vi "show_message.vi"(6 "display time (ms)":i32=5000, 7 "Icon (None)":i32(ring) items=["None", "Info", "Warning", "Error"], 8 "error in (no error)":errorcluster, 9 "Text":string, 10 "Title":string, 11 "BalloonNotifier in":refnum<class "BalloonNotifier.lvclass">) -> (0 "error out":errorcluster, 3 "BalloonNotifier out":refnum<class "BalloonNotifier.lvclass">)   [LabVIEW 2010, in "BalloonNotifier.lvclass"]
uses:
  BalloonNotifier.lvclass
  BalloonNotifier.lvclass/BalloonNotifier.ctl
  System.Windows.Forms
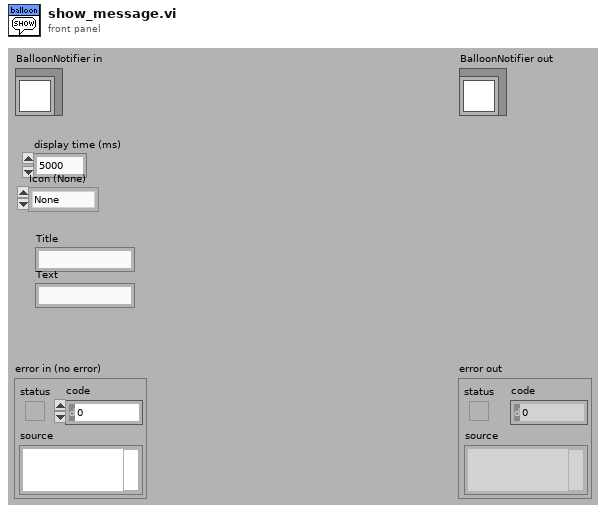
[diagram p1: front panel]
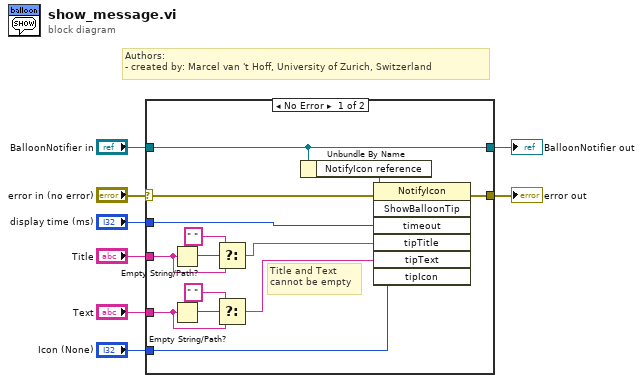
[diagram p0: block diagram]
diagram:
  # "Authors: \n- created by: Marcel van 't Hoff, University of Zurich, Switzerland"
  n1 = case shown="No Error" "error in (no error)" {
    selector: "error in (no error)" -> [w11 w24]
    tunnel: "display time (ms)" -> [w22 _]
    tunnel: [w21 w24] -> w7
    tunnel: "Icon (None)" -> [w20 _]
    tunnel: "Title" -> [w18 _]
    tunnel: "Text" -> [w13 _]
    tunnel: "BalloonNotifier in" -> [w9 w23]
    tunnel: [w9 w23] -> w1
    frame No Error {
      # "Title and Text\ncannot be empty"
      n2 = Empty String/Path?(string/path=w18) -> (empty?=w19:bool)
      n3 = Empty String/Path?(string/path=w13) -> (empty?=w14:bool)
      n4 = Select(t=" ", s=w19, f=w18) -> (s? t:f=w16:string)
      n5 = Select(t=" ", s=w14, f=w13) -> (s? t:f=w12:string)
      n6 = Unbundle By Name(w9) -> ("NotifyIcon reference"=w10:refnum<k24>)
      n7 = invoke class="NotifyIcon" method="ShowBalloonTip"(reference=w10, error in=w11, "timeout"=w22, "tipTitle"=w16, "tipText"=w12, "tipIcon"=w20) -> (error out=w21:errorcluster)  [unwired: 1 in, 6 out]
    }
    frame Error {
    }
  }
  "error out" <- w7
  "BalloonNotifier out" <- w1
